vi "Read LED INI File.vi"(8 "error in":errorcluster) -> (0 "error out":errorcluster, 2 "data":T1={"TestPlan"={"Current Consumption"=FALSE, "Emission Spectrum"=FALSE}, "Instruments"={"Resistor 1"=1600.0, "Resistor 2"=0.0, "Resistor 3"=0.0}, "Limits"={"Current 1"=0.0, "Current 2"=0.0, "Current 3"=0.0, "Tolerance"=0.0, "Wavelength"=0.0}, "Settings"={"VLED 1"=0.0, "VLED 2"=0.0, "VLED 3"=0.0, "Source V"=0.0, "Result Path"=path ""}} {"Settings"."Source V" format="%#_g V"; "Settings"."VLED 3" format="%#_g V"; "Settings"."VLED 2" format="%#_g V"; "Settings"."VLED 1" format="%#f V"; "Limits"."Wavelength" format="%#_g nm"; "Limits"."Tolerance" format="%#_g %"; "Limits"."Current 3" format="%#_g  mA"; "Limits"."Current 2" format="%#_g  mA"; "Limits"."Current 1" format="%#_g mA"; "Instruments"."Resistor 3" format="%#_g ohm"; "Instruments"."Resistor 2" format="%#_g ohm"; "Instruments"."Resistor 1" format="%#f ohm"})   [LabVIEW 2018, in "LED Control Module.lvlib" / "LED INI File.lvlib"]
uses:
  LED INI File.lvlib
  INI File Control.ctl
  Public Controls/LVS Testplan.ctl
  Public Controls/LVS Instruments.ctl
  Public Controls/LVS Limits.ctl
  Public Controls/LVS Settings.ctl
  <vilib>/Utility/config.llb/NI_LVConfig.lvlib
  LED Control Module.lvlib
panel:
  in  "LED INI Settings":T1 {"Settings"."Source V" format="%#_g V"; "Settings"."VLED 3" format="%#_g V"; "Settings"."VLED 2" format="%#_g V"; "Settings"."VLED 1" format="%#f V"; "Limits"."Wavelength" format="%#_g nm"; "Limits"."Tolerance" format="%#_g %"; "Limits"."Current 3" format="%#_g  mA"; "Limits"."Current 2" format="%#_g  mA"; "Limits"."Current 1" format="%#_g mA"; "Instruments"."Resistor 3" format="%#_g ohm"; "Instruments"."Resistor 2" format="%#_g ohm"; "Instruments"."Resistor 1" format="%#f ohm"}
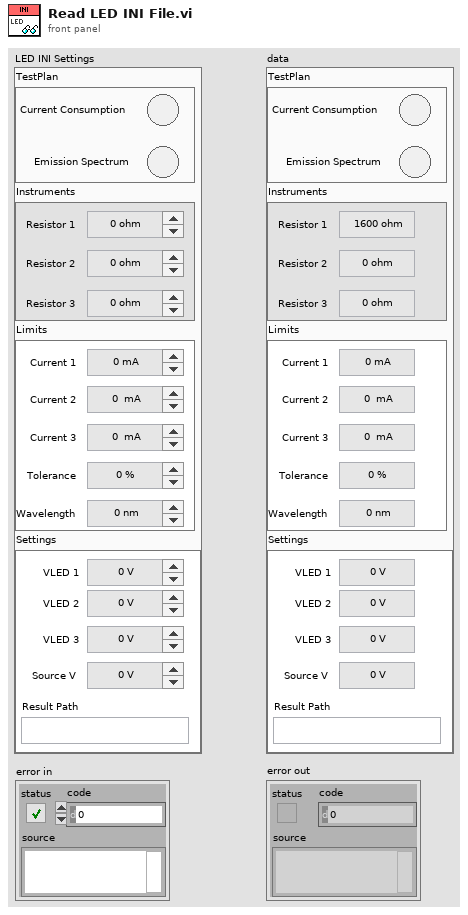
[diagram p1: front panel]
types:
  T1 = typedef "LED Control Module.lvlib/LED INI File.lvlib/INI File Control.ctl" = cluster{"TestPlan":T2, "Instruments":T3, "Limits":T4, "Settings":T5}
  T2 = typedef "LED Control Module.lvlib/LVS Testplan.ctl" = cluster{"Current Consumption":bool, "Emission Spectrum":bool}
  T3 = typedef "LED Control Module.lvlib/LVS Instruments.ctl" = cluster{"Resistor 1":dbl, "Resistor 2":dbl, "Resistor 3":dbl}
  T4 = typedef "LED Control Module.lvlib/LVS Limits.ctl" = cluster{"Current 1":dbl, "Current 2":dbl, "Current 3":dbl, "Tolerance":dbl, "Wavelength":dbl}
  T5 = typedef "LED Control Module.lvlib/LVS Settings.ctl" = cluster{"VLED 1":dbl, "VLED 2":dbl, "VLED 3":dbl, "Source V":dbl, "Result Path":path}
  T6 = enum32{"invalid app kind", "Development System", "Run Time System", "Student Edition", "Embedded LabVIEW", "Evaluation", "Custom"}
  T7 = typedef "NI_LVConfig.lvlib/Config Data RefNum.ctl" = refnum<k1>
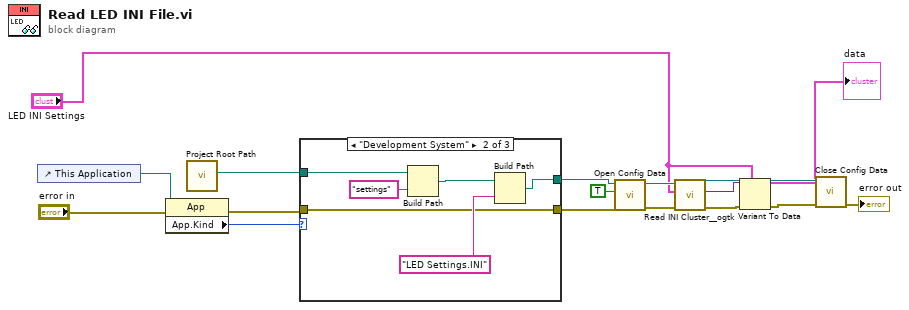
[diagram p0: block diagram]
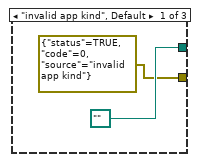
[diagram p2: hidden frame]
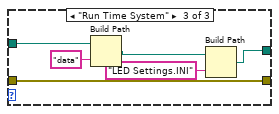
[diagram p3: hidden frame]
diagram:
  n1 = control-ref of="This Application"() -> (w17:refnum<vi>)
  n2 = property class="App"(reference=w17, error in="error in") -> (error out=w9:errorcluster, "App.Kind"=w16:T6)  [unwired: 1 out]
  n3 = call "Project Root Path.vi"() -> ("stripped path"=w15:path)  [unwired: 11 in]
  n4 = case shown="\"Development System\"" w16 {
    tunnel: w15 -> [_ w25 w31]
    tunnel: [path "" ("appended path") w21 w27] -> w12
    tunnel: [errorcluster {"status"=TRUE, "code"=0, "source"="invalid app kind"} ("error out") w20 w26] -> w10
    tunnel: w9 -> [_ w20 w26]
    frame "invalid app kind", Default {
    }
    frame "Development System" {
      n5 = Build Path(base path=w25, name or relative path="settings") -> (appended path=w23:path)
      n6 = Build Path(base path=w23, name or relative path="LED Settings.INI") -> (appended path=w21:path)
    }
    frame "Run Time System" {
      n7 = Build Path(base path=w31, name or relative path="data") -> (appended path=w28:path)
      n8 = Build Path(base path=w28, name or relative path="LED Settings.INI") -> (appended path=w27:path)
    }
  }
  n9 = call <vilib>:"Open Config Data.vi"("error in (no error)"=w10, "create file if necessary (T)"=TRUE, "configuration file path"=w12) -> ("error out"=w14:errorcluster, "refnum"=w13:T7)  [unwired: 6 in, 1 out]
  n10 = call <userlib>:"Read INI Cluster__ogtk.vi"("error in (no error)"=w14, "INI Fomatted Cluster Type"="LED INI Settings", "refnum"=w13) -> ("error out"=w5:errorcluster, "INI Fomatted Cluster"=w3:variant, "dup refnum"=w7:T7)  [unwired: 4 in, 2 out]
  n11 = Variant To Data(error in=w5, type="LED INI Settings", Variant=w3) -> (data=→"data":T1, error out=w4:errorcluster)
  n12 = call <vilib>:"Close Config Data.vi"("error in (no error)"=w4, "refnum"=w7) -> ("error out"=→"error out":errorcluster)  [unwired: 8 in, 1 out]
